vi "CRYCurve Library Error Message.vi"(7 "sAction":string, 8 "Type":enum16{"Curves", "Values", "Results", "WFM"}(ring)=enum."Results", 9 "sData":string, 10 "sOption":string, 11 "error IO":errorcluster) -> ()   [LabVIEW 2013]
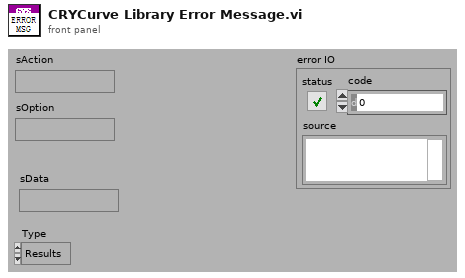
[diagram p1: front panel]
types:
  T1 = enum16{"OK", "Yes", "YesNo", "YesNoCancel", "ReplaceAppend"}
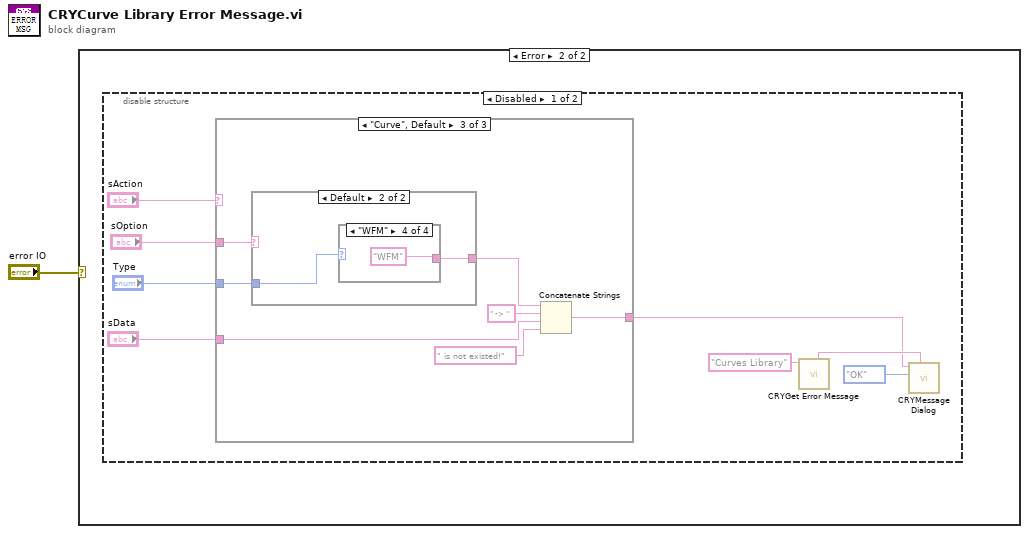
[diagram p0: block diagram]
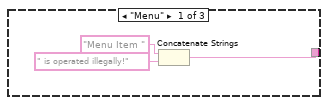
[diagram p3: hidden frame]
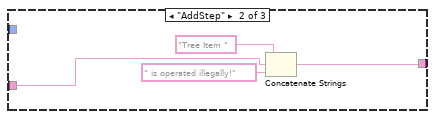
[diagram p4: hidden frame]
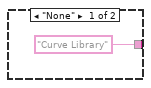
[diagram p5: hidden frame]
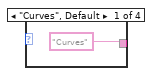
[diagram p6: hidden frame]
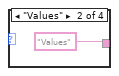
[diagram p7: hidden frame]
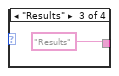
[diagram p8: hidden frame]
diagram:
  n1 = case shown="Error" "error IO" {
    frame No Error {
    }
    frame Error {
      n2 = disable-structure shown="Disabled" {
        frame Disabled {
          n3 = case shown="\"Curve\", Default" "sAction" {
            tunnel: "sData" -> [_ w14 w21]
            tunnel: [w11 w15 w19] -> w5
            tunnel: "sOption" -> [_ _ w18]
            tunnel: "Type" -> [_ _ w17]
            frame "Menu" {
              n4 = Concatenate Strings("Menu Item " ("string"), " is operated illegally!" ("string")) -> (w11:string)
            }
            frame "AddStep" {
              n5 = Concatenate Strings("Tree Item " ("string"), w14, " is operated illegally!" ("string")) -> (w15:string)
            }
            frame "Curve", Default {
              n6 = case shown="Default" w18 {
                tunnel: ["Curve Library" ("Kind") w26] -> w23
                tunnel: w17 -> [_ w25]
                frame "None" {
                }
                frame Default {
                  n7 = case shown="\"WFM\"" w25 {
                    tunnel: ["Curves" ("Kind") "Values" ("Kind") "Results" ("Kind") "WFM" ("Kind")] -> w26
                    frame "Curves", Default {
                    }
                    frame "Values" {
                    }
                    frame "Results" {
                    }
                    frame "WFM" {
                    }
                  }
                }
              }
              n8 = Concatenate Strings(w23, " -> " ("string"), w21, " is not existed!" ("string")) -> (w19:string)
            }
          }
          n9 = call "CRYGet Error Message.vi"("Kind"="Curves Library") -> ("Window Title"=w8:string)  [unwired: 5 in, 5 out]
          n10 = call "CRYMessage Dialog.vi"("Window Title"=w8, "YesNoCancel"=T1."OK", "Message Content"=w5) -> ()  [unwired: 7 in, 2 out]
        }
        frame Enabled {
        }
      }
    }
  }
